vi "SIMPLE_Ping.vi"() -> ()   [LabVIEW 2016]
uses:
  <vilib>/Instr/_visa.llb/VISA Set IO Buffer Mask.ctl
  <vilib>/Utility/miscctls.llb/LVPointTypeDef.ctl
  <vilib>/Instr/_visa.llb/VISA Configure Serial Port (Instr).vi
  GEN_2.lvlib
panel:
  out "Version":T1 {"DRV Ver" format="%x"; "HW Ver" format="%x"; "FW Ver" format="%x"}
  out "ERROR":u8
  in  "ID":u8=1 format="%x"
  in  "Baud rate":u32=8000000
  in  "Com port":refnum<visa-resource-name>="COM8"
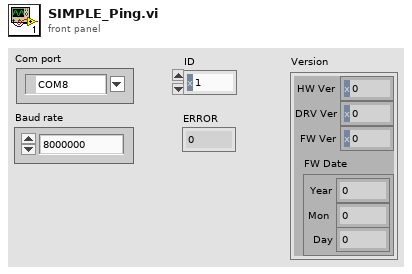
[diagram p1: front panel]
types:
  T1 = cluster{"HW Ver":u8, "DRV Ver":u8, "FW Ver":u16, "FW Date":cluster{"Year":u32, "Mon":u32, "Day":u32}}
  T2 = typedef "LVPointTypeDef.ctl" = cluster{"Horizontal":i16, "Vertical":i16}
  T3 = typedef "VISA Set IO Buffer Mask.ctl" = u16
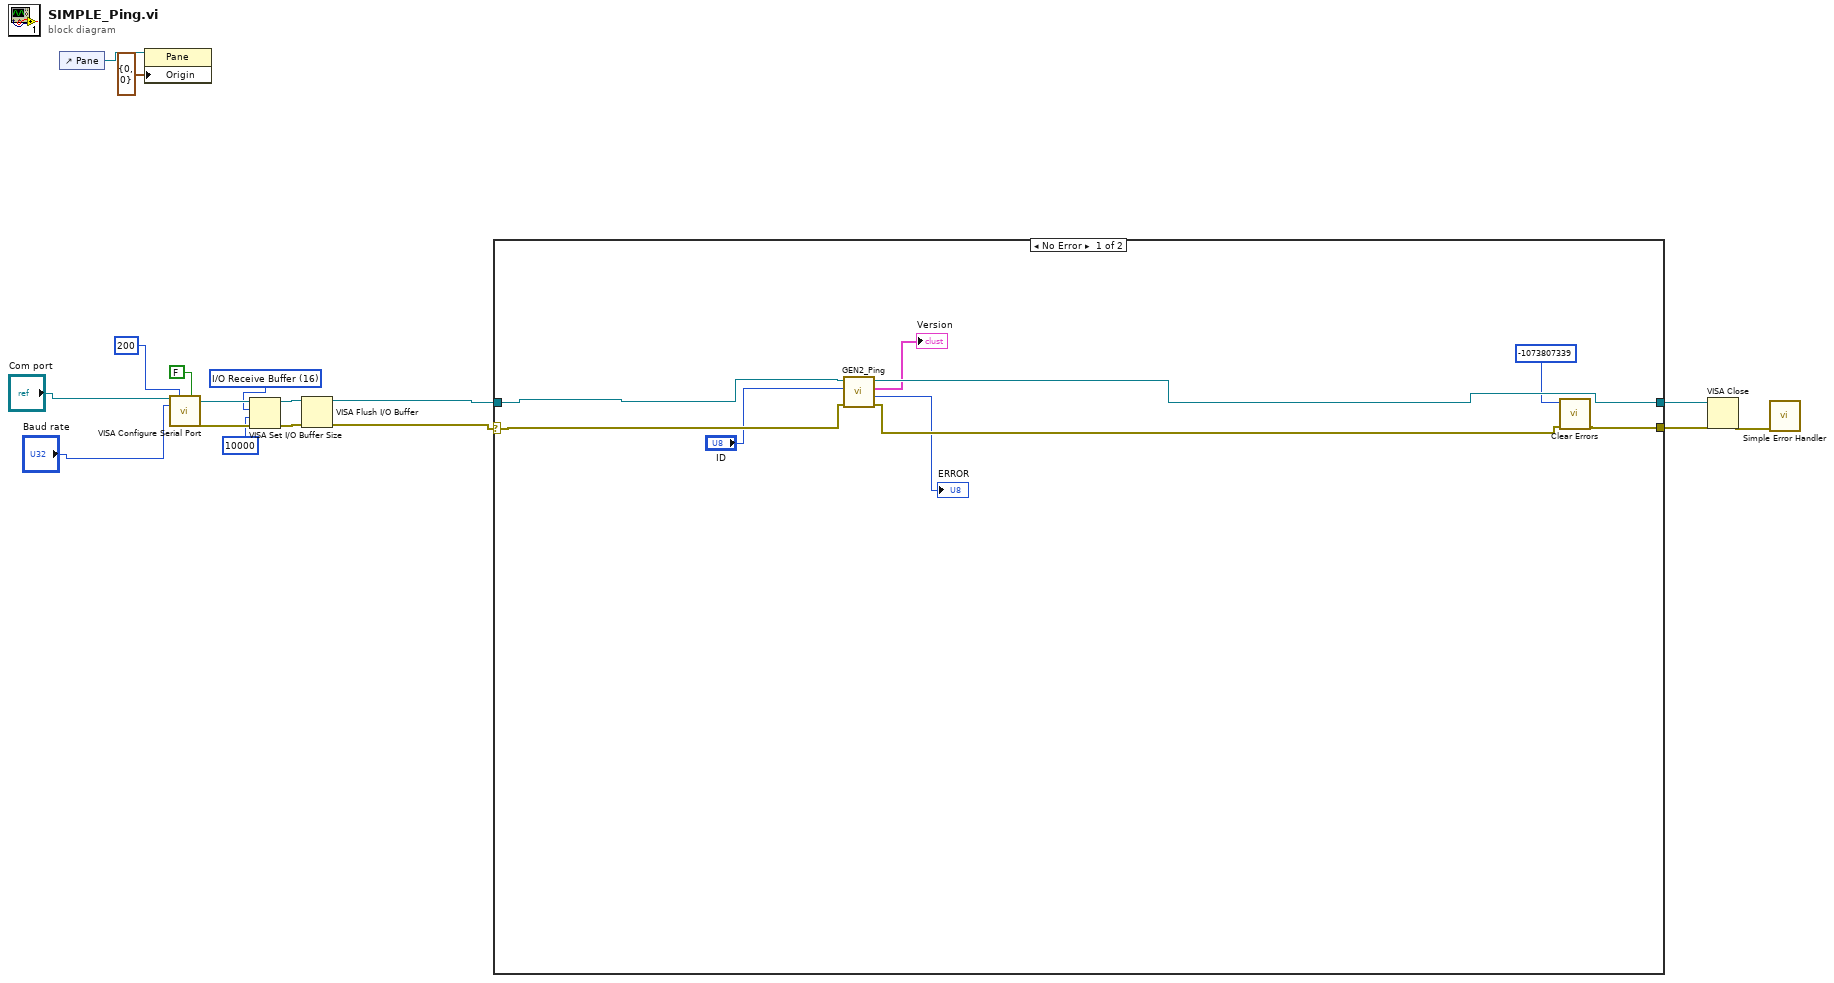
[diagram p0: block diagram]
diagram:
  w9 = T3 16 items=["I/O Receive Buffer"=16, "I/O Transmit Buffer"=32, "I/O Receive and Transmit Buffer"=48] ("Mask")
  n1 = control-ref of="Pane"() -> (w4:refnum<vi>)
  n2 = property class="Pane"(reference=w4, "Origin"=T2 {"Horizontal"=0, "Vertical"=0}) -> ()  [unwired: 1 in, 2 out]
  n3 = call-poly "VISA Configure Serial Port"("VISA resource name"="Com port", "timeout (10sec)"=u32 200, "Enable Termination\nChar (T)"=FALSE ("Enable Termination\nChar (T)"), "baud rate (9600)"="Baud rate") -> ("VISA resource name out"=w10:refnum<visa-resource-name>, "error out"=w13:errorcluster)  [unwired: 10 in]
  n4 = VISA Set I/O Buffer Size(VISA resource name=w10, mask (16)=w9, size (4096)=u32 10000, error in (no error)=w13) -> (VISA resource name out=w11:refnum<visa-resource-name>, error out=w12:errorcluster)
  n5 = VISA Flush I/O Buffer(VISA resource name=w11, error in (no error)=w12) -> (VISA resource name out=w1:refnum<visa-resource-name>, error out=w2:errorcluster)  [unwired: 1 in]
  n6 = case shown="No Error" w2 {
    selector: w2 -> [w23 w27]
    tunnel: [w26 w27] -> w17
    tunnel: w1 -> [w25 w28]
    tunnel: [w24 w28] -> w15
    frame No Error {
      n7 = call "GEN2_Ping.vi"("error in (no error)"=w23, "ID"="ID", "VISA Refnum in"=w25) -> ("error out"=w21:errorcluster, "ERROR"=→"ERROR":u8, "Version"=→"Version":T1, "VISA Refnum out"=w24:refnum<visa-resource-name>)  [unwired: 5 in]
      n8 = call <vilib>:"Clear Errors.vi"("error in (no error)"=w21, "specific error code to clear (0: all)"=-1073807339) -> ("error out"=w26:errorcluster)  [unwired: 4 in, 1 out]
    }
    frame Error {
    }
  }
  n9 = VISA Close(VISA resource name=w15, error in (no error)=w17) -> (error out=w7:errorcluster)
  n10 = call <vilib>:"Simple Error Handler.vi"("error in (no error)"=w7) -> ()  [unwired: 4 in, 5 out]
